vi "Multi-Device Tx and Rx Streaming Time (Host).vi"() -> ()   [LabVIEW 2015]
doc: "This template is for the Simple NI-USRP Streaming design, a design that shows the basics of streaming data to and from an NI USRP-294x/295x device. Refer to the block diagram for more information about how to use this template."
uses:
  <vilib>/Utility/error.llb/DialogType.ctl
  <vilib>/userdefined/Silver/nirio_resource_slv.ctl
  SubVIs/Start Trigger.ctl
panel:
  in  "config tab":enum32{"Tx Configuration", "Rx Configuration"}(tab)
  in  "tx config":T2={"rf enable 0"=TRUE, "rf config 0"={"antenna"="TX1", "frequency"=2000000000.0, "lo frequency"=-1.0, "level"=0.0}, "rf enable 1"=TRUE, "rf config 1"={"antenna"="TX1", "frequency"=2000000000.0, "lo frequency"=-1.0, "level"=0.0}, "transfer mode"=enum."Finite", "sample rate"=10000000.0, "number of samples"=8192, "start trigger"=enum."Future Time Event", "tone frequency"=100000.0} {"tone frequency" format="%#.3pHz"; "sample rate" format="%#.3pS/s"; "rf config 0"."level" format="%#_gdBm"; "rf config 0"."lo frequency" format="%#.3pHz"; "rf config 0"."frequency" format="%#.3pHz"; "rf config 1"."level" format="%#_gdBm"; "rf config 1"."lo frequency" format="%#.3pHz"; "rf config 1"."frequency" format="%#.3pHz"}
  in  "rx config":T3={"rf enable 0"=TRUE, "rf config 0"={"antenna"="RX2", "frequency"=2000000000.0, "lo frequency"=-1.0, "level"=0.0}, "rf enable 1"=TRUE, "rf config 1"={"antenna"="RX2", "frequency"=2000000000.0, "lo frequency"=-1.0, "level"=0.0}, "transfer mode"=enum."Finite", "sample rate"=10000000.0, "number of samples"=8192, "start trigger"=enum."Future Time Event"} {"sample rate" format="%#.3pS/s"; "rf config 1"."level" format="%#_gdBm"; "rf config 1"."lo frequency" format="%#.3pHz"; "rf config 1"."frequency" format="%#.3pHz"; "rf config 0"."level" format="%#_gdBm"; "rf config 0"."lo frequency" format="%#.3pHz"; "rf config 0"."frequency" format="%#.3pHz"}
  out "acquiring":bool caption="Acquiring"
  in  "tx.stop":bool
  out "generating":bool caption="Generating"
  in  "USRP RIO devices":T4[](array[typedef])=["RIO0", "RIO1"] caption="USRP RIO Devices"
  in  "reference frequency source":string(combo)="REF IN" caption="Reference Frequency Source"
  in  "indicator tab":T5(tab)
  out "tx.waveform":waveform(dbl)[](graph) caption="Output Waveform"
  out "power spectrum":cluster{"f0":dbl, "df":dbl, "magnitude":dbl[]}[](graph) caption="Power Spectrum"
  out "power level":dbl[][](graph) caption="Power Level"
  out "iq data":waveform(dbl)[](graph) caption="I & Q Data"
  out "tx.coerced config":T6(array[cluster]) caption="Tx" {"coerced sample rates" format="%#.3pS/s"; "coerced levels" format="%#.3gdBm"; "coerced lo frequencies" format="%#.3pHz"; "coerced frequencies" format="%#.3pHz"}
  out "rx.coerced config":T6(array[cluster]) caption="Rx" {"coerced sample rates" format="%#.3pS/s"; "coerced levels" format="%#.3gdBm"; "coerced lo frequencies" format="%#.3pHz"; "coerced frequencies" format="%#.3pHz"}
  in  "rx.stop":bool
  # "This template is for the Simple NI-USRP Streaming design, a design that shows the basics of streaming data on an NI 294x/295x device. See the block diagram for more information on how to use this template."
  # "Multi-Device Tx and Rx Streaming with Time"
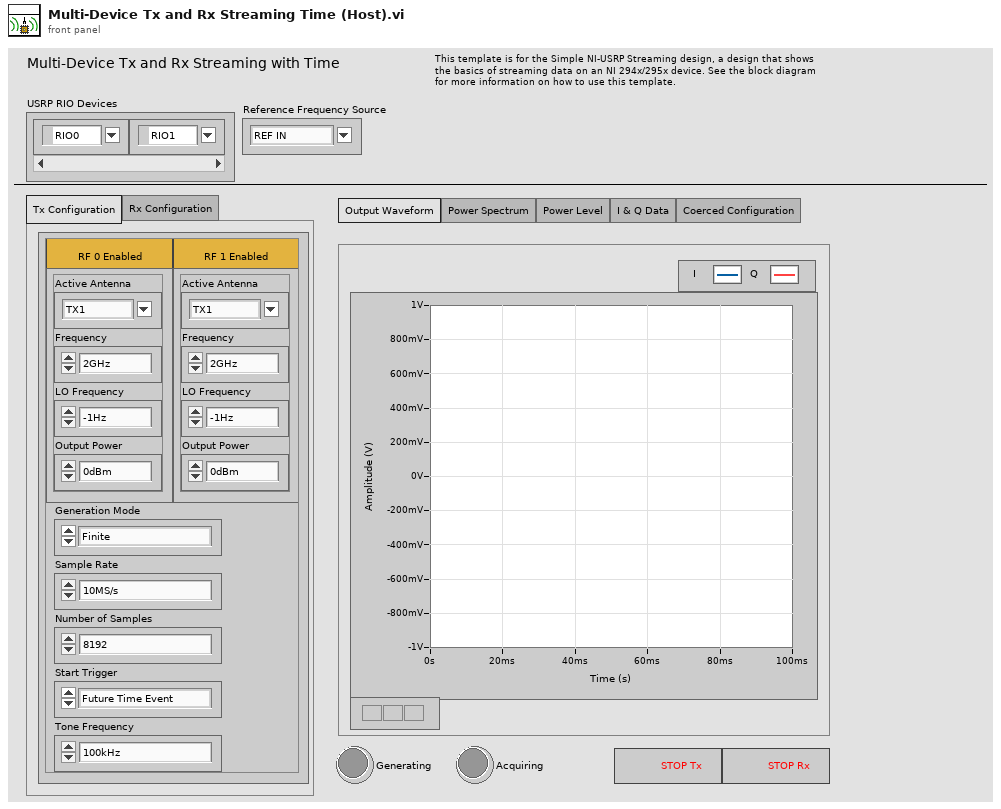
[diagram p1: front panel]
types:
  T1 = typedef "Start Trigger.ctl" = enum8{"Software", "Digital Edge", "Rx Start Trigger", "Tx Start Trigger", "Immediate", "Future Time Event"}
  T2 = cluster{"rf enable 0":bool, "rf config 0":cluster{"antenna":string, "frequency":dbl, "lo frequency":dbl, "level":dbl}, "rf enable 1":bool, "rf config 1":cluster{"antenna":string, "frequency":dbl, "lo frequency":dbl, "level":dbl}, "transfer mode":enum16{"Finite", "Continuous"}, "sample rate":dbl, "number of samples":u32, "start trigger":T1, "tone frequency":dbl}
  T3 = cluster{"rf enable 0":bool, "rf config 0":cluster{"antenna":string, "frequency":dbl, "lo frequency":dbl, "level":dbl}, "rf enable 1":bool, "rf config 1":cluster{"antenna":string, "frequency":dbl, "lo frequency":dbl, "level":dbl}, "transfer mode":enum16{"Finite", "Continuous"}, "sample rate":dbl, "number of samples":u32, "start trigger":T1}
  T4 = typedef "nirio_resource_slv.ctl" = tag
  T5 = enum32{"Output Waveform", "Power Spectrum", "Power Level", "I & Q Data", "Coerced Configuration"}
  T6 = cluster{"coerced frequencies":dbl[], "coerced lo frequencies":dbl[], "coerced levels":dbl[], "coerced sample rates":dbl[]}[]
  T7 = typedef "DialogType.ctl" = u16
  T8 = cluster{"rx config":cluster{"rf enable 0":bool, "rf config 0":cluster{"antenna":string, "frequency":dbl, "lo frequency":dbl, "level":dbl}, "rf enable 1":bool, "rf config 1":cluster{"antenna":string, "frequency":dbl, "lo frequency":dbl, "level":dbl}, "transfer mode":enum16{"Finite", "Continuous"}, "sample rate":dbl, "number of samples":u32, "start trigger":T1}, "reference frequency source":string, "rx.enabled channels":string[], "vertical range":dbl[], "rx.coerced configurations":cluster{"coerced frequencies":dbl[], "coerced lo frequencies":dbl[], "coerced levels":dbl[], "coerced sample rates":dbl[]}}
  T9 = cluster{"tx config":cluster{"rf enable 0":bool, "rf config 0":cluster{"antenna":string, "frequency":dbl, "lo frequency":dbl, "level":dbl}, "rf enable 1":bool, "rf config 1":cluster{"antenna":string, "frequency":dbl, "lo frequency":dbl, "level":dbl}, "transfer mode":enum16{"Finite", "Continuous"}, "sample rate":dbl, "number of samples":u32, "start trigger":T1, "tone frequency":dbl}, "reference frequency source":string, "tx.enabled channels":string[], "I":i16[], "Q":i16[], "tx.coerced configurations":cluster{"coerced frequencies":dbl[], "coerced lo frequencies":dbl[], "coerced levels":dbl[], "coerced sample rates":dbl[]}}
  T10 = typedef "niUsrpRio Config v1 Host.lvlib/niUsrpRio Session.ctl" = cluster{"FPGA Interface":refnum<k20>, "RIO Interface Number":u32, "Data Clock Rate":u32, "FPGA Data Clock Rate":u32, "Global Settings Register Bus":T11, "Radio 0 Settings Register Bus":T11, "Radio 1 Settings Register Bus":T11, "Radio Settings Bus Semaphore":T12, "DB Queues":T13[], "Characterization Data Valid?":bool, "EEPROM Header":T14, "Device Data Header":T15, "EEPROM Characterization Header":T16, "Characterization Data":T17[], "FPGA Current Version":u32, "FPGA Oldest Compatible Version":u32, "Fixed Logic Current Version":u32, "Fixed Logic Oldest Compatible Version":u32, "FPGA Radio Settings Bus Current Version":u32, "FPGA Radio Settings Bus Oldest Compatible Version":u32, "FPGA Board Config Current Version":u32, "FPGA Board Config Oldest Compatible Version":u32, "Daughterboard Clock Rate":u32}
  T11 = typedef "niInstr Register Bus v0 Host.lvlib/Register Bus Session.ctl" = refnum<queue>
  T12 = typedef "Semaphore RefNum" = refnum<k1>
  T13 = typedef "niUsrpRio Config v1 Host.lvlib/DB Queue Reference.ctl" = refnum<queue>
  T14 = typedef "niUsrpRio Config v1 Host.lvlib/EEPROM Header.ctl" = cluster{"Checksum":u32, "Product Code":u16, "Hardware Current Version":u16, "Hardware Oldest Compatible Version":u16, "EEPROM Map Current Version":u16, "EEPROM Map Oldest Compatible Version":u16, "User Password":string, "Pointer to Factory Header":u32, "Pointer to User Header":u32, "Recommended Interval":u16, "Number of Reserved Bytes":i32, "Number of Daughterboards":u8, "Daughterboard IDs":u16[], "Daughterboard Serial Numbers":string[]}
  T15 = typedef "niUsrpRio Config v1 Host.lvlib/EEPROM Device Data Header.ctl" = cluster{"Checksum":u32, "Number of Channels":u8, "Number of Gain Settings":u16[], "Pointer to Characterization Data":u32[], "Number of Reserved Bytes":i32, "Number of Frequencies":u16[]}
  T16 = typedef "niUsrpRio Config v1 Host.lvlib/EEPROM Characterization Header.ctl" = cluster{"Checksum":u32, "Date":timestamp, "Temperature":sgl, "Misc. Info":string, "Pointer to Device Data Header":u32, "Number of Reserved Bytes":i32}
  T17 = typedef "niUsrpRio Config v1 Host.lvlib/Characterization Data.ctl" = cluster{"Gains[dB]":dbl[], "Frequencies [Hz]":dbl[], "IQ Imbalance Table":T18[], "Measured Gains[dB]":dbl[][]}
  T18 = typedef "niUsrpRio Config v1 Host.lvlib/IQ Imbalance.ctl" = cluster{"Gain Imbalance [linear]":dbl, "Phase Imbalance [radians]":dbl, "Offset":cdb}
  T19 = cluster{"coerced frequencies":dbl[], "coerced lo frequencies":dbl[], "coerced levels":dbl[], "coerced sample rates":dbl[]}
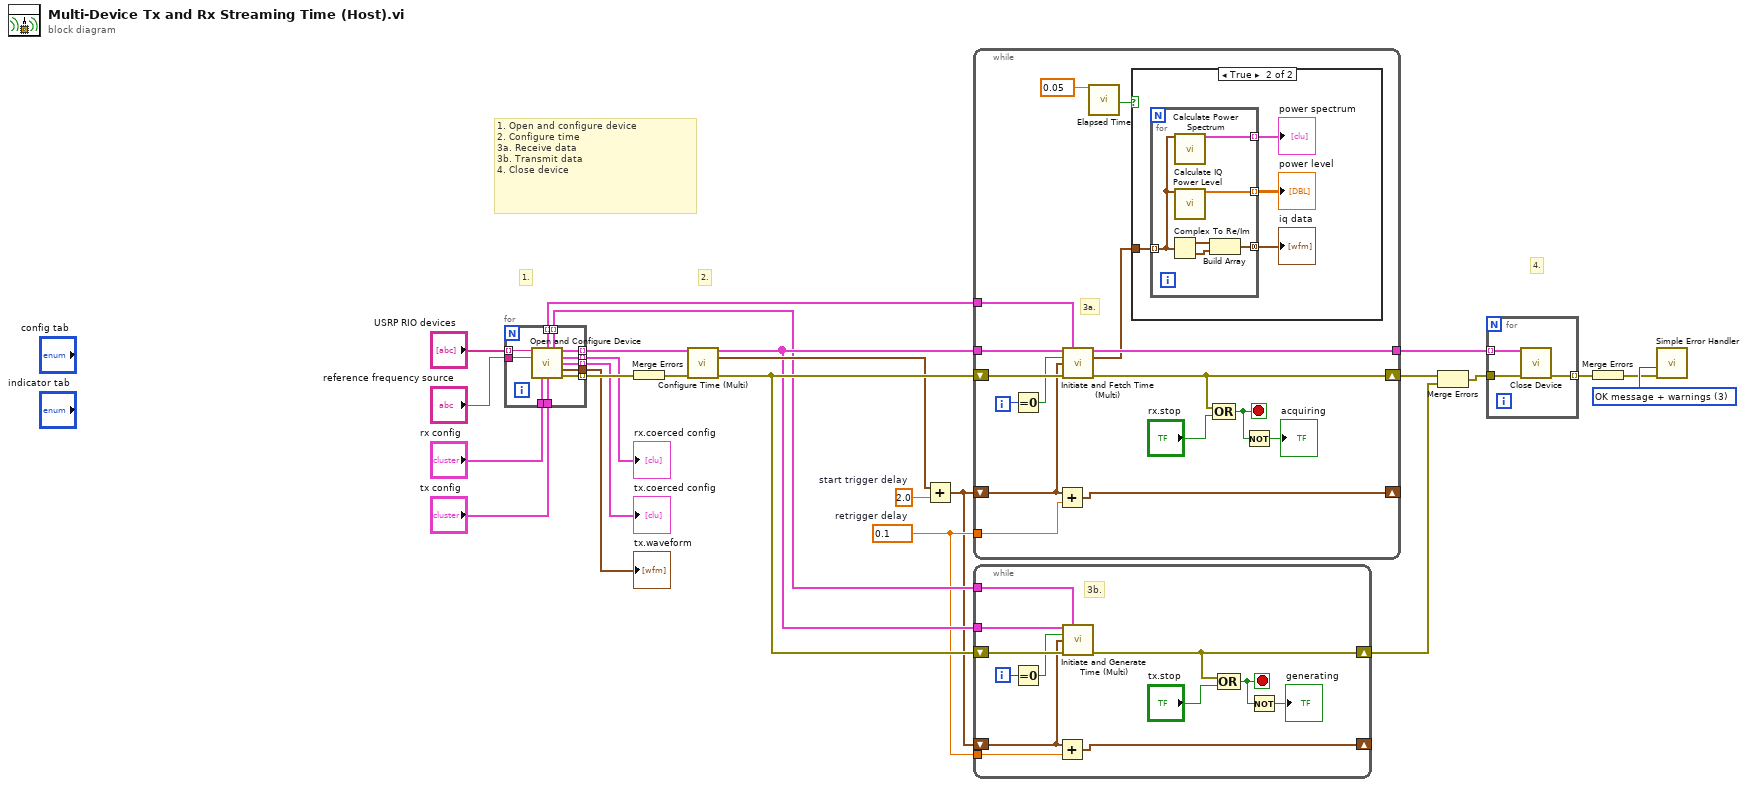
[diagram p0: block diagram]
diagram:
  w3 = 2.0  # start trigger delay
  w2 = 0.1  # retrigger delay
  w22 = T7 3 items=["no dialog", "OK message", "continue or stop message", "OK message + warnings", "continue/stop + warnings"] ("type of dialog (OK msg:1)")
  # "4."
  # "2."
  # "1. Open and configure device\n2. Configure time\n3a. Receive data\n3b. Transmit data\n4. Close device"
  # "1."
  n1 = for {
    tunnel: [w36] -> w23 mode=indexing
    tunnel: [w35] -> w20 mode=indexing
    tunnel: "rx config" -> [w34]
    tunnel: "tx config" -> [w33]
    tunnel: "reference frequency source" -> [w32]
    tunnel: [w31] -> w9 mode=indexing
    tunnel: [w30] -> w8 mode=indexing
    tunnel: [w29] -> w15
    tunnel: [w28] -> w14 mode=indexing
    tunnel: [w27] -> w12 mode=indexing
    tunnel: "USRP RIO devices" -> [w26] mode=indexing
    n2 = call "Open and Configure Device.vi"("USRP RIO Device"=w26, "reference frequency source"=w32, "rx config"=w34, "tx config"=w33) -> ("rx channels"=w35:T8, "tx channels"=w27:T9, "niUsrpRio Session (out)"=w28:T10, "rx.coerced configurations"=w31:T19, "tx.coerced configurations"=w30:T19, "tx.output waveform"=w29:waveform(dbl)[], "error out"=w36:errorcluster)  [unwired: 5 in]
  }
  "tx.waveform" <- w15
  "tx.coerced config" <- w8
  "rx.coerced config" <- w9
  n3 = Merge Errors(w23) -> (w4:errorcluster)
  n4 = call "Configure Time (Multi).vi"("niUsrpRio Sessions"=w14, "error in"=w4) -> ("niUsrpRio Sessions (out)"=w13:T10[], "time"=w24:timestamp, "error out"=w25:errorcluster)  [unwired: 11 in]
  n5 = Add(x=w24, y=w3) -> (x+y=w1:timestamp)
  n6 = while {
    tunnel: w13 -> [w50]
    tunnel: [w47] -> w5
    tunnel: w20 -> [w44]
    shift-right: [w48] -> w6
    shift-left: w25 -> [w51]
    tunnel: w2 -> [w38]
    shift-right: [w37] -> _
    shift-left: w1 -> [w39]
    i -> [w49]
    stop <- w45 stop-if-true
    # "3a."
    # "Acquire and Fetch a waveform"
    n7 = Equal To 0?(x=w49) -> (x = 0?=w40:bool)
    n8 = Add(x=w39, y=w38) -> (x+y=w37:timestamp)
    n9 = call "Initiate and Fetch Time (Multi).vi"("niUsrpRio Sessions"=w50, "rx channels"=w44, "first iteration"=w40, "start trigger time"=w39, "error in"=w51) -> ("niUsrpRio Sessions (out)"=w47:T10[], "complex baseband data"=w41:waveform(cdb)[], "error out"=w48:errorcluster)  [unwired: 8 in]
    n10 = call "Elapsed Time"("Time Target (s)"=0.05 ("retrigger delay")) -> ("Time has Elapsed"=w42:bool)  [unwired: 11 in, 7 out]
    n11 = case shown="True" w42 {
      tunnel: w41 -> [_ w56]
      frame False {
      }
      frame True {
        n12 = for {
          tunnel: [w60] -> w55 mode=concatenating
          tunnel: [w59] -> w54 mode=indexing
          tunnel: [w58] -> w53 mode=indexing
          tunnel: w56 -> [w57] mode=indexing
          n13 = Complex To Re/Im(x + iy=w57) -> (x=w62:waveform(dbl), y=w61:waveform(dbl))
          n14 = call "Calculate Power Spectrum.vi"("waveform"=w57) -> ("power spectrum (dBm)"=w58:cluster{"f0":dbl, "df":dbl, "magnitude":dbl[]})  [unwired: 14 in]
          n15 = call "Calculate IQ Power Level.vi"("iq data"=w57) -> ("power level (dBm)"=w59:dbl[])  [unwired: 14 in]
          n16 = Build Array(w62, w61) -> (w60:waveform(dbl)[])
        }
        "power level" <- w54
        "power spectrum" <- w53
        "iq data" <- w55
      }
    }
    n17 = Compound Arithmetic op=OR(w48, "rx.stop") -> (w45:bool)
    n18 = Not(x=w45) -> (.not. x?=→"acquiring":bool)
  }
  n19 = while {
    tunnel: w13 -> [w72]
    tunnel: w12 -> [w67]
    shift-right: [w70] -> w7
    shift-left: w25 -> [w71]
    tunnel: w2 -> [w65]
    shift-right: [w63] -> _
    shift-left: w1 -> [w64]
    i -> [w69]
    stop <- w68 stop-if-true
    # "3b."
    # "Acquire and Fetch a waveform"
    n20 = Equal To 0?(x=w69) -> (x = 0?=w66:bool)
    n21 = Add(x=w64, y=w65) -> (x+y=w63:timestamp)
    n22 = call "Initiate and Generate Time (Multi).vi"("niUsrpRio Sessions"=w72, "tx channels"=w67, "first iteration"=w66, "start trigger time"=w64, "error in"=w71) -> ("error out"=w70:errorcluster)  [unwired: 9 in, 1 out]
    n23 = Compound Arithmetic op=OR(w70, "tx.stop") -> (w68:bool)
    n24 = Not(x=w68) -> (.not. x?=→"generating":bool)
  }
  n25 = Merge Errors(w6, w7) -> (w19:errorcluster)
  n26 = for {
    tunnel: w5 -> [w75] mode=indexing
    tunnel: w19 -> [w76]
    tunnel: [w77] -> w21 mode=indexing
    n27 = call "Close Device.vi"("niUsrpRio Session"=w75, "error in"=w76) -> ("error out"=w77:errorcluster)  [unwired: 13 in]
  }
  n28 = Merge Errors(w21) -> (w10:errorcluster)
  n29 = call <vilib>:"Simple Error Handler.vi"("type of dialog (OK msg:1)"=w22, "error in (no error)"=w10) -> ()  [unwired: 3 in, 5 out]
